vi "MovePos3.vi"(7 "In Contact in":bool, 10 "Position 3":bool, 11 "UiDefinition 2":T1) -> (3 "In Contact out":bool)   [LabVIEW 2020]
uses:
  UIReferences.ctl
  C:/Users/User/Desktop/Automation/CurrentVersion/LabviewDXFViewer/bin/Release/LabviewDXFViewer.exe
  LabviewDXFViewer/bin/Release/LabviewDXFViewer.exe
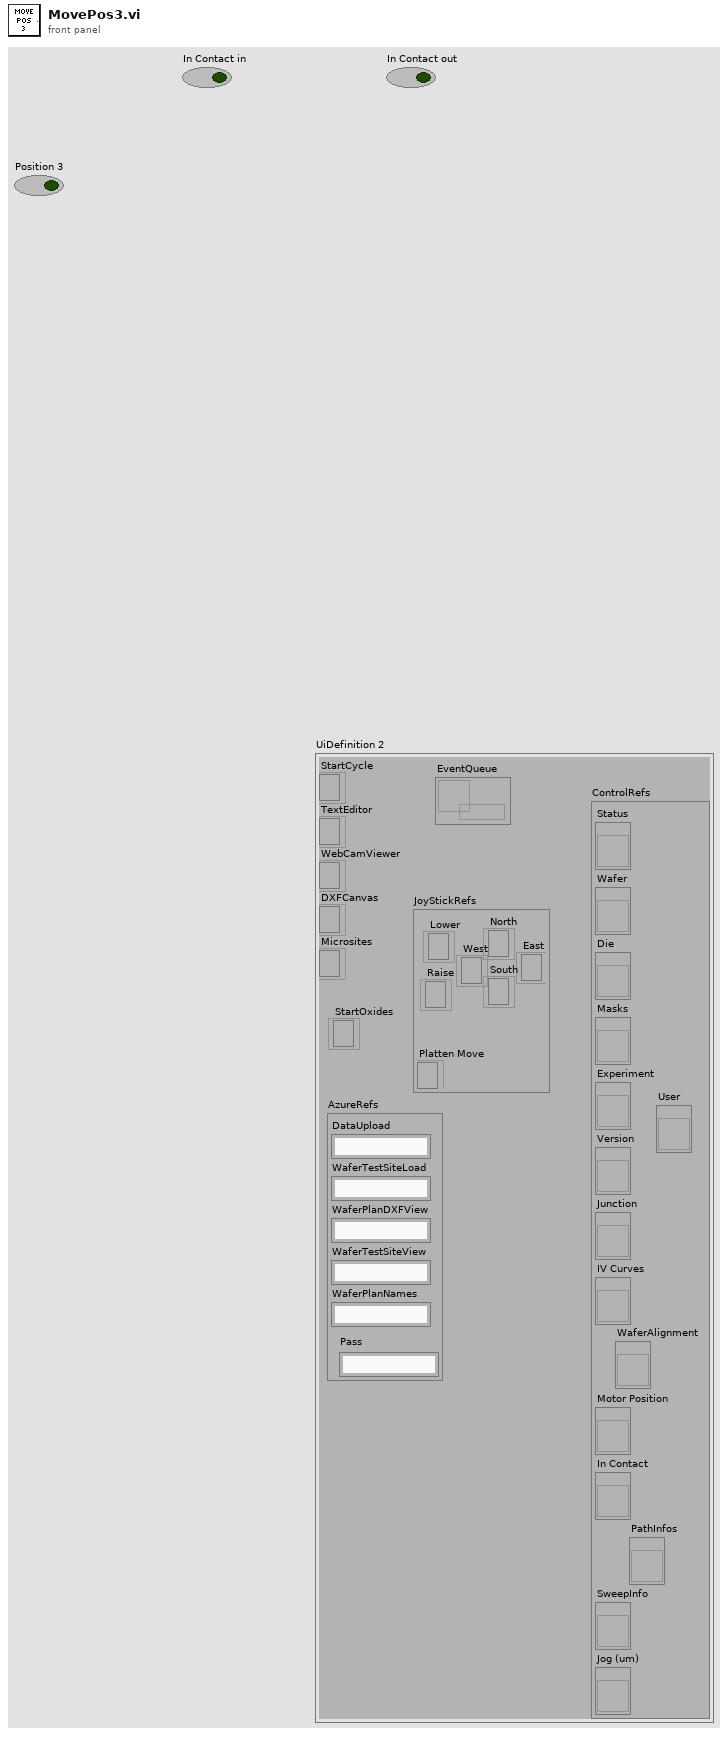
[diagram p1: front panel]
types:
  T1 = typedef "UIReferences.ctl" = cluster{"StartCycle":refnum<k24>, "TextEditor":refnum<k24>, "WebCamViewer":refnum<k24>, "DXFCanvas":refnum<k24>, "Microsites":refnum<k24>, "JoyStickRefs":cluster{"North":refnum<k24>, "Lower":refnum<k24>, "Raise":refnum<k24>, "Platten Move":refnum<k24>, "West":refnum<k24>, "East":refnum<k24>, "South":refnum<k24>}, "AzureRefs":cluster{"DataUpload":string, "WaferTestSiteLoad":string, "WaferPlanDXFView":string, "WaferTestSiteView":string, "WaferPlanNames":string, "Pass":string}, "ControlRefs":cluster{"Status":refnum<vi>, "Wafer":refnum<vi>, "Die":refnum<vi>, "Masks":refnum<vi>, "Experiment":refnum<vi>, "Version":refnum<vi>, "Junction":refnum<vi>, "IV Curves":refnum<vi>, "Motor Position":refnum<vi>, "In Contact":refnum<vi>, "SweepInfo":refnum<vi>, "Jog (um)":refnum<vi>, "PathInfos":refnum<vi>, "User":refnum<vi>, "WaferAlignment":refnum<vi>}, "EventQueue":refnum<queue>, "StartOxides":refnum<k24>}
  T2 = typedef "WaferAlignmentType.ctl" = cluster{"Wafer Units to microns":dbl, "Rotation Misalign":dbl[], "Scale Misalign":dbl, "Steps Per micron":dbl, "Position 1":i32[], "Position 2":i32[], "Lift Distance":i32, "Position 3":i32[], "Jog Height":i32}
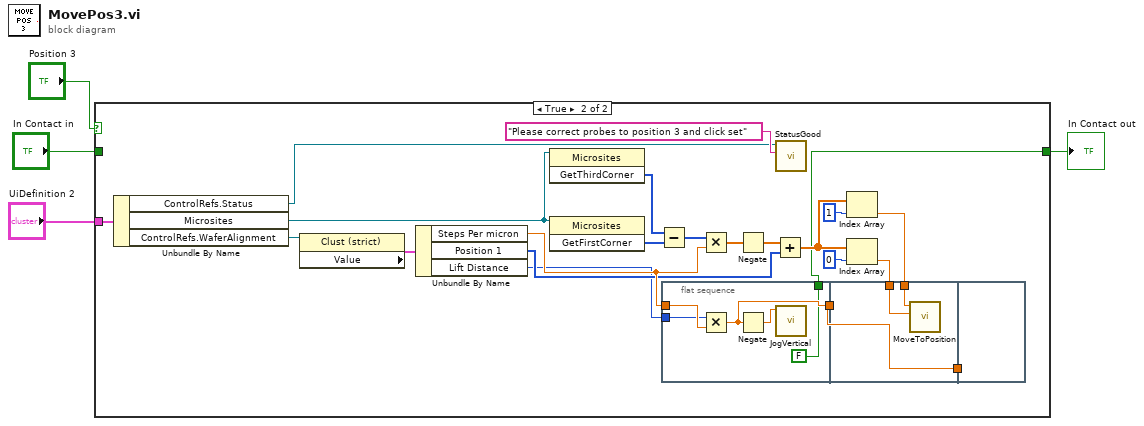
[diagram p0: block diagram]
diagram:
  n1 = case shown="True" "Position 3" {
    tunnel: [w5 w11] -> w3
    tunnel: "In Contact in" -> [w5 _]
    tunnel: "UiDefinition 2" -> [_ w8]
    frame False {
    }
    frame True {
      n2 = Unbundle By Name(w8) -> ("ControlRefs.Status"=w6:refnum<vi>, "Microsites"=w7:refnum<k24>, "ControlRefs.WaferAlignment"=w10:refnum<vi>)
      n3 = property class="Clust (strict)"(reference=w10) -> ("Value"=w9:T2)  [unwired: 1 in, 2 out]
      n4 = Unbundle By Name(w9) -> ("Steps Per micron"=w14:dbl, "Position 1"=w13:i32[], "Lift Distance"=w12:i32)
      n5 = invoke class="Microsites" method="GetThirdCorner"(reference=w7) -> ("GetThirdCorner"=w27:i32[])  [unwired: 2 in, 2 out]
      n6 = invoke class="Microsites" method="GetFirstCorner"(reference=w7) -> ("GetFirstCorner"=w25:i32[])  [unwired: 2 in, 2 out]
      n7 = Subtract(x=w27, y=w25) -> (x-y=w26:i32[])
      n8 = flat-sequence {
        tunnel: w14 -> [w31]
        tunnel: [w30] -> w20
        tunnel: w12 -> [w29]
        tunnel: [FALSE ("In Contact")] -> w11
        tunnel: w23 -> [w35]
        tunnel: w22 -> [w34]
        tunnel: [w33] -> w21
        tunnel: w20 -> [w33]
        tunnel: w21 -> [_]
        frame #0 {
          n9 = Multiply(x=w29, y=w31) -> (x*y=w30:dbl)
          n10 = Negate(x=w30) -> (-x=w32:dbl)
          n11 = call "JogVertical.vi"("Numeric"=w32) -> ()  [unwired: 11 in]
        }
        frame #1 {
          n12 = call "MoveToPosition.vi"("Y"=w35, "X"=w34) -> ()  [unwired: 10 in]
        }
        frame #2 {
        }
      }
      n13 = Multiply(x=w26, y=w14) -> (x*y=w24:dbl[])
      n14 = Negate(x=w24) -> (-x=w16:dbl[])
      n15 = Add(x=w16, y=w13) -> (x+y=w17:dbl[])
      n16 = call "StatusGood.vi"("Text.Text"="Please correct probes to position 3 and click set" ("Status"), "String in"=w6) -> ()  [unwired: 10 in]
      n17 = Index Array(array=w17, index=1) -> (element=w22:dbl)
      n18 = Index Array(array=w17, index=0) -> (element=w23:dbl)
    }
  }
  "In Contact out" <- w3
